vi "Read Data.vi"(8 "error in (no error)":errorcluster, 11 "Vec3d Class in":refnum<class "Vec3d.lvclass">) -> (0 "error out":errorcluster, 2 "Data":cluster{"X":dbl, "Y":dbl, "Z":dbl}, 3 "Vec3d Class out":refnum<class "Vec3d.lvclass">)   [LabVIEW 2024, in "Vec3d.lvclass"]
uses:
  Vec3d.lvclass
  Vec3d.lvclass/Vec3d.ctl
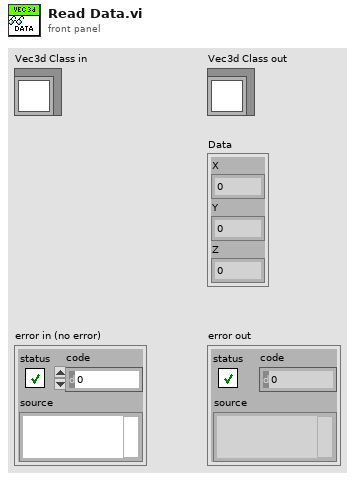
[diagram p1: front panel]
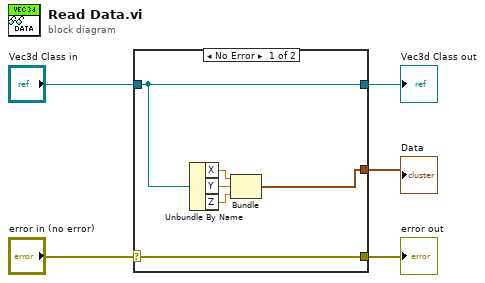
[diagram p0: block diagram]
diagram:
  n1 = case shown="No Error" "error in (no error)" {
    selector: "error in (no error)" -> [w11 w12]
    tunnel: [w11 w12] -> w4
    tunnel: [w10 w13] -> w2
    tunnel: "Vec3d Class in" -> [w10 w13]
    tunnel: [w6 _] -> w1
    frame No Error {
      n2 = Unbundle By Name(w10) -> ("X"=w9:dbl, "Y"=w8:dbl, "Z"=w7:dbl)
      n3 = Bundle("X"=w9, "Y"=w8, "Z"=w7) -> (w6:cluster{"X":dbl, "Y":dbl, "Z":dbl})  [unwired: 1 in]
    }
    frame Error {
    }
  }
  "error out" <- w4
  "Vec3d Class out" <- w2
  "Data" <- w1
